vi "T7 Auto Target Bit Mask KAG.vi"(1 "bit mask":bool[](array[boolean])=[TRUE, FALSE, FALSE, FALSE, FALSE, FALSE, FALSE, FALSE] caption="1 : Send to Ethernet 702 sockets") -> (0 "Auto Target":u32=1)   [LabVIEW 2022 SP3]
doc: "Auto Target controls where data will be sent. Value is a bitmask. \n\nbit 0 : 1 = Send to Ethernet 702 sockets\nbit 1 : 1 = Send to USB\nbit 4 : 1 = Command-Response mode\nAll other bits are reserved\n\nAdditional Note Re: bit 4\nbit 4 sets how data is sent to its destination. A zero value will set the stream data output to \"Spontaneous Mode\" which means the T7 will stream it to the host automatically without a Modbus command request. A value of 1 will set the stream data output to \"Command-Response Mode\""
panel:
  out "bit mask":u32=1 format="%.0b"
  # "Auto Target controls where data will be sent. Value is a bitmask. \n\nbit 0 : 1 = Send to Ethernet 702 sockets\nbit 1 : 1 = Send to USB\nbit 4 : 1 = Command-Response mode\nAll other bits are reserved\n\nAdditional Note Re: bit 4\nbit 4 sets how data is sent to its destination. A zero value will set the stream data output to \"Spontaneous Mode\" which means the T7 will stream it to the host automatically without a Modbus command request. A value of 1 will set the stream data output to \"Command-Response Mode\""
  # "bit 0"
  # "1 : Send to Ethernet 702 Sockets"
  # "bit 1"
  # "1 : Send to USB"
  # "bit 2"
  # "bit 3"
  # "bit 4"
  # "1 : Command-Response Mode"
  # "bit 5"
  # "bit 6"
  # "bit 7"
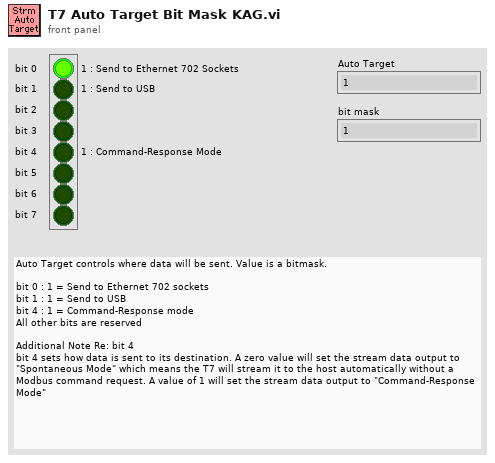
[diagram p1: front panel]
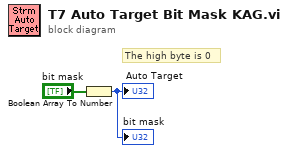
[diagram p0: block diagram]
diagram:
  # "The high byte is 0"
  n1 = Boolean Array To Number(Boolean array="bit mask") -> (number=→"Auto Target" →"bit mask":u32)
